vi "Write measurement that is requesting hardware.vi"(10 "Measurement Name":string, 11 "Find Compatible Hardware for Measurement Msg in":refnum<class "Find Compatible Hardware for Measurement Msg.lvclass">) -> (3 "Find Compatible Hardware for Measurement Msg out":refnum<class "Find Compatible Hardware for Measurement Msg.lvclass">)   [LabVIEW 2017, in "Controller Actor.lvlib" / "Find Compatible Hardware for Measurement Msg.lvclass"]
uses:
  Find Compatible Hardware for Measurement Msg.lvclass
  Find Compatible Hardware for Measurement Msg.lvclass/Find Compatible Hardware for Measurement Msg.ctl
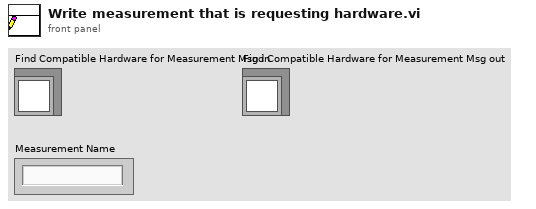
[diagram p1: front panel]
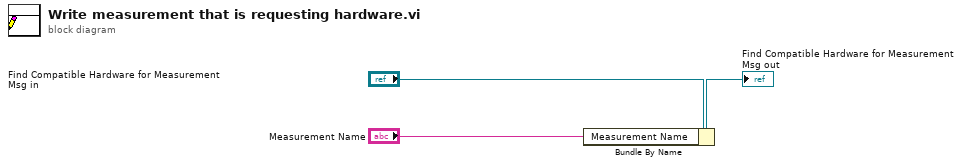
[diagram p0: block diagram]
diagram:
  n1 = Bundle By Name(cluster="Find Compatible Hardware for Measurement Msg in", "Measurement Name"="Measurement Name") -> (→"Find Compatible Hardware for Measurement Msg out":refnum<class "Find Compatible Hardware for Measurement Msg.lvclass">)
